vi "Lorentzian function dispersive.vi"(3 "output control":T1, 4 "data":variant, 5 "X":dbl[](array[numeric]), 6 "params":dbl[](array[numeric])) -> (0 "error out":errorcluster, 1 "f'(X,a)":dbl[][](array[numeric]), 2 "f(X,a)":dbl[](array[numeric]))   [LabVIEW 2015]
doc: "Given a set of x-values and parameters (x0, gamma), outputs the resulting Lorentzian curve.\n\n(Connector panel is in a form that allows this VI to be passed to the Nonlinear Curve Fit.vi.)"
uses:
  <vilib>/gmath/NumericalOptimization/LM_output select.ctl
  <vilib>/gmath/NI_Gmath.lvlib
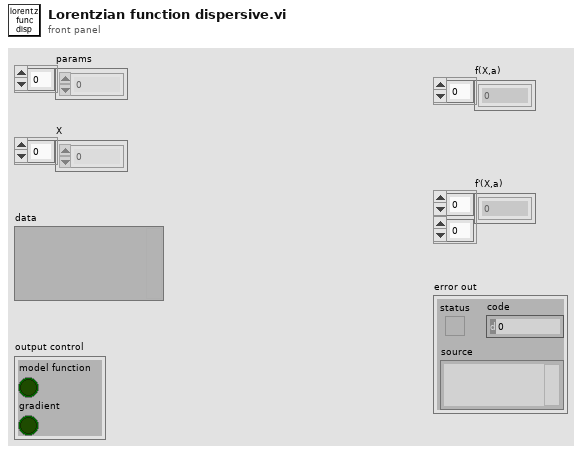
[diagram p1: front panel]
types:
  T1 = typedef "NI_Gmath.lvlib/LM_output select.ctl" = cluster{"model function":bool, "gradient":bool}
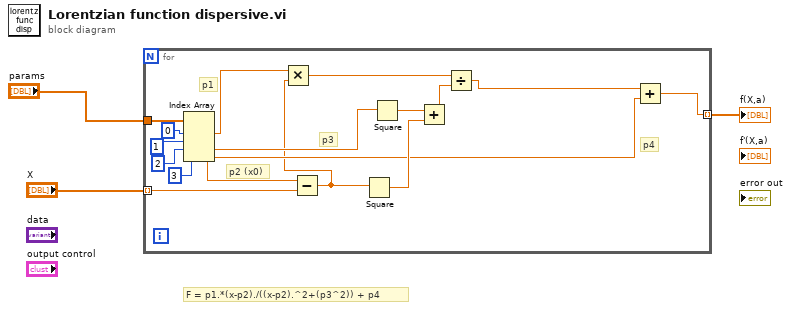
[diagram p0: block diagram]
diagram:
  # "F = p1.*(x-p2)./((x-p2).^2+(p3^2)) + p4"
  n1 = for {
    tunnel: "params" -> [w17]
    tunnel: "X" -> [w16] mode=indexing
    tunnel: [w9] -> w1 mode=indexing
    # "p3"
    # "p4"
    # "p2 (x0)"
    # "p1"
    n2 = Index Array(array=w17, index #1=0 ("index (col)"), index #2=1 ("disabled index (col)"), index #3=2 ("index"), index #4=3 ("index")) -> (element #1=w11:dbl, element #2=w18:dbl, element #3=w8:dbl, element #4=w10:dbl)
    n3 = Subtract(x=w18, y=w16) -> (x-y=w4:dbl)
    n4 = Multiply(x=w11, y=w4) -> (x*y=w5:dbl)
    n5 = Square(x=w4) -> (x^2=w19:dbl)
    n6 = Square(x=w8) -> (x^2=w20:dbl)
    n7 = Add(x=w20, y=w19) -> (x+y=w7:dbl)
    n8 = Divide(x=w5, y=w7) -> (x/y=w6:dbl)
    n9 = Add(x=w6, y=w10) -> (x+y=w9:dbl)
  }
  "f(X,a)" <- w1
